vi "Escape String for Windows.vi"(8 "error in":errorcluster, 11 "String in":string) -> (0 "error out":errorcluster, 3 "String out":string)   [LabVIEW 2025, in "Process Executor.lvclass"]
doc: "Prepares a single command-line argument for safe use on the Windows command line.\n\nThe VI escapes double quotes and backslashes according to Windows parsing rules when quoting is required, ensuring that the argument is interpreted correctly by the target process."
uses:
  Process Executor.lvclass
  <vilib>/regexp/Match Regular Expression.xnode
  Process Executor.lvclass/Process Executor.ctl
panel:
  # "\"C:\\Path\\\\\\\"Test\\\"\""
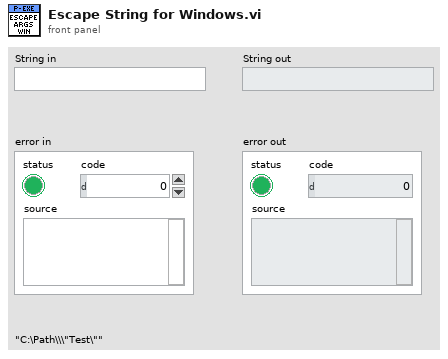
[diagram p1: front panel]
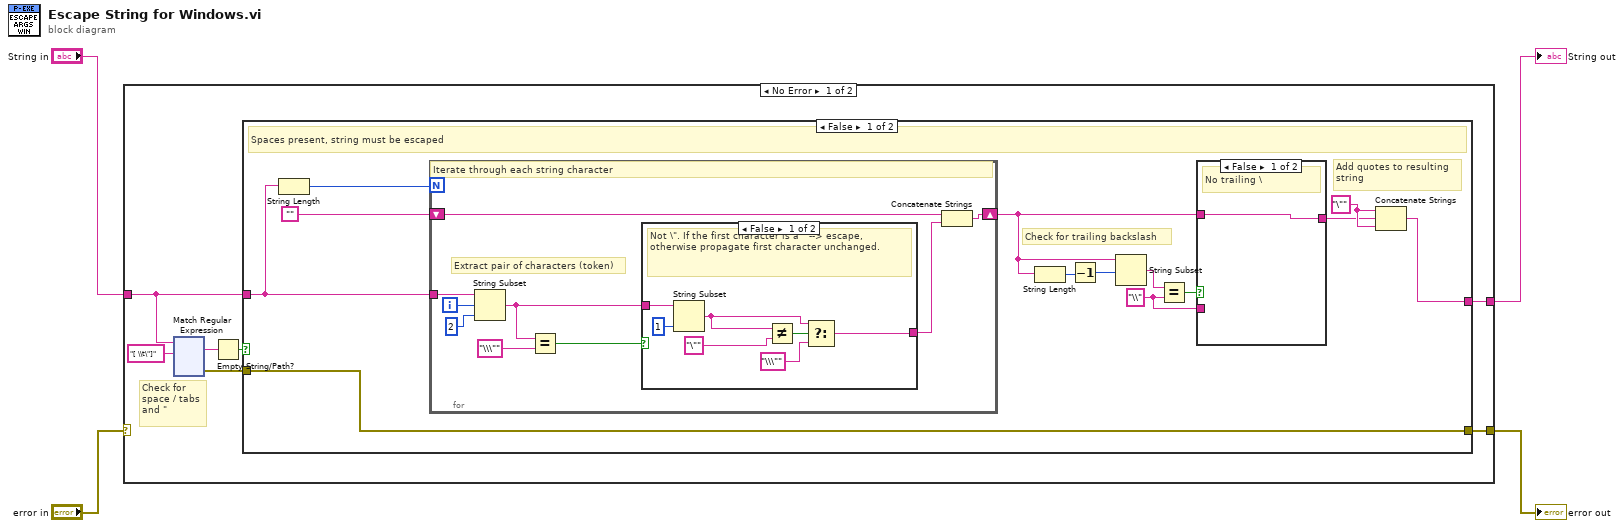
[diagram p0: block diagram]
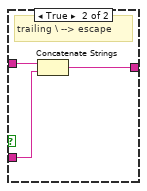
[diagram p2: hidden frame]
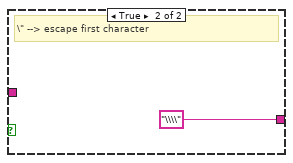
[diagram p3: hidden frame]
diagram:
  n1 = case shown="No Error" "error in" {
    selector: "error in" -> [_ w165]
    tunnel: "String in" -> [w9 _]
    tunnel: [w10 w165] -> w3
    tunnel: [w5 _] -> w1
    frame No Error {
      # "Check for\nspace / tabs\nand \""
      n2 = xnode ("Match Regular Expression")("input string"=w9, "regular expression"="[ \\t\"]") -> ("whole match"=w7:string, "error out"=w11:errorcluster)  [unwired: 4 in, 3 out]
      n3 = Empty String/Path?(string/path=w7) -> (empty?=w6:bool)
      n4 = case shown="False" w6 {
        tunnel: w9 -> [w19 w46]
        tunnel: w11 -> [w24 w47]
        tunnel: [w24 w47] -> w10
        tunnel: [w20 w46] -> w5
        frame False {
          w13 = "\\" ("y")
          w21 = "\""
          # "Add quotes to resulting\nstring"
          # "Check for trailing backslash"
          # "Spaces present, string must be escaped"
          n5 = String Length(string=w19) -> (length=w23:i32)
          n6 = for {
            N: w23 -> [_]
            tunnel: w19 -> [w33]
            shift-right: [w35] -> w14
            shift-left: "" ("Empty String Constant") -> [w37]
            i -> [w32]
            # "Extract pair of characters (token)"
            # "Iterate through each string character"
            n7 = String Subset(string=w33, offset (0)=w32, length (rest)=2 ("length (rest)")) -> (substring=w31:string)
            n8 = Equal?(x=w31, y="\\\"") -> (x = y?=w29:bool)
            n9 = case shown="False" w29 {
              tunnel: [w40 "\\\\"] -> w36
              tunnel: w31 -> [w44 _]
              frame False {
                # "Not \\\". If the first character is a \" --> escape, otherwise propagate first character unchanged."
                n10 = String Subset(string=w44, length (rest)=1 ("length (rest)")) -> (substring=w38:string)  [unwired: 1 in]
                n11 = Not Equal?(x=w38, y="\"") -> (x != y?=w41:bool)
                n12 = Select(t=w38, s=w41, f="\\\"" ("y")) -> (s? t:f=w40:string)
              }
              frame True {
                # "\\\" --> escape first character"
              }
            }
            n13 = Concatenate Strings(w37, w36) -> (w35:string)
          }
          n14 = String Length(string=w14) -> (length=w18:i32)
          n15 = Decrement(x=w18) -> (x-1=w17:i32)
          n16 = String Subset(string=w14, offset (0)=w17) -> (substring=w16:string)  [unwired: 1 in]
          n17 = Equal?(x=w16, y=w13) -> (x = y?=w15:bool)
          n18 = case shown="False" w15 {
            tunnel: w14 -> [w25 w28]
            tunnel: w13 -> [_ w27]
            tunnel: [w25 w26] -> w12
            frame False {
              # "No trailing \\"
            }
            frame True {
              # "trailing \\ --> escape"
              n19 = Concatenate Strings(w28, w27) -> (w26:string)
            }
          }
          n20 = Concatenate Strings(w21, w12, w21) -> (w20:string)
        }
        frame True {
          # "No spaces present, no escaping needed."
        }
      }
    }
    frame Error {
      # "Pass error without further action"
    }
  }
  "String out" <- w1
  "error out" <- w3
